vi "LaserCal-Update Sequence (PT).vi"(0 "Stimulus (I-O)":T3, 5 "Runtime State":T2, 7 "SCL Element":T1, 9 "Start?":bool, 11 "error in (no error)":errorcluster) -> (15 "error out":errorcluster)   [LabVIEW 2015]
uses:
  Typedefs/LaserCal-Meter Stimulus.ctl
  Typedefs/LaserCal-Control Mode.ctl
  Typedefs/LaserCal-Meter Runtime State.ctl
  Typedefs/LaserCal-StimConList Element.ctl
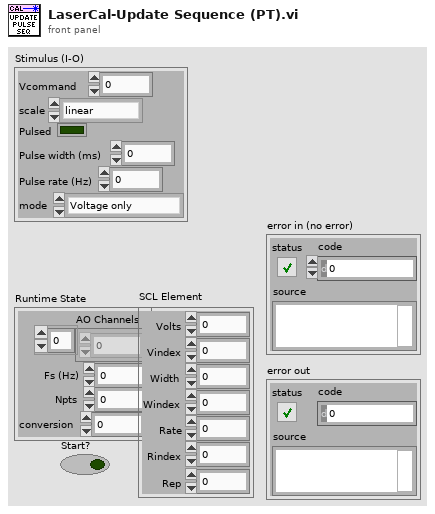
[diagram p1: front panel]
types:
  T1 = typedef "LaserCal-StimConList Element.ctl" = cluster{"Volts":dbl, "Vindex":i32, "Width":dbl, "Windex":i32, "Rate":dbl, "Rindex":i32, "Rep":i32}
  T2 = typedef "LaserCal-Meter Runtime State.ctl" = cluster{"AO Channels":i32[], "Fs (Hz)":dbl, "Npts":i32, "conversion":dbl}
  T3 = typedef "LaserCal-Meter Stimulus.ctl" = cluster{"Vcommand":dbl, "scale":enum16{"linear", "dB"}, "Pulsed":bool, "Pulse width (ms)":dbl, "Pulse rate (Hz)":dbl, "mode":T4}
  T4 = typedef "LaserCal-Control Mode.ctl" = enum16{"Voltage only", "Voltage + Enable"}
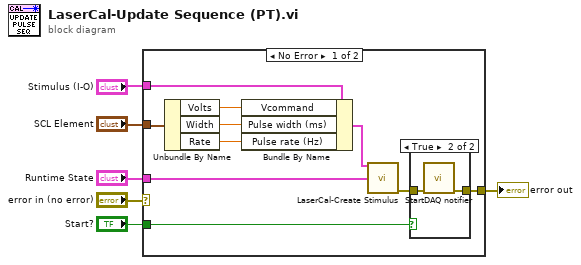
[diagram p0: block diagram]
diagram:
  n1 = case shown="No Error" "error in (no error)" {
    selector: "error in (no error)" -> [_ w20]
    tunnel: [w12 w20] -> w4
    tunnel: "Runtime State" -> [w15 _]
    tunnel: "Stimulus (I-O)" -> [w14 _]
    tunnel: "Start?" -> [w11 _]
    tunnel: "SCL Element" -> [w10 _]
    frame No Error {
      n2 = Unbundle By Name(w10) -> ("Volts"=w9:dbl, "Width"=w8:dbl, "Rate"=w7:dbl)
      n3 = Bundle By Name(cluster=w14, "Vcommand"=w9, "Pulse width (ms)"=w8, "Pulse rate (Hz)"=w7) -> (w13:T3)
      n4 = call "LaserCal-Create Stimulus.vi"("Stimulus"=w13, "Runtime State"=w15) -> ("error out"=w16:errorcluster)  [unwired: 11 in, 2 out]
      n5 = case shown="True" w11 {
        tunnel: w16 -> [w17 w19]
        tunnel: [w17 w18] -> w12
        frame False {
        }
        frame True {
          n6 = call "StartDAQ notifier.vi"("error in (no error)"=w19) -> ("error out"=w18:errorcluster)  [unwired: 6 in]
        }
      }
    }
    frame Error {
    }
  }
  "error out" <- w4
